vi "SC10_get_baud.vi"() -> ()   [LabVIEW 2010]
panel:
  out "substring":string
  in  "VISA resource name":refnum<visa-resource-name>
  out "VISA resource name out":refnum<visa-resource-name>
  out "read buffer":string
  out "return count 2":u32
  out "return count":u32
  out "error out":errorcluster
  in  "error in (no error)":errorcluster
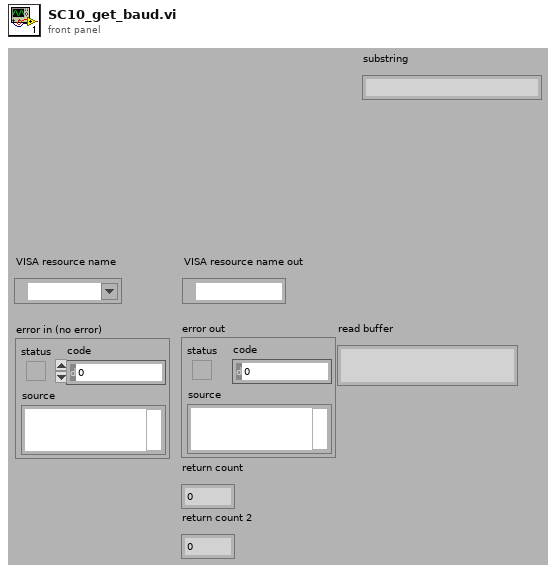
[diagram p1: front panel]
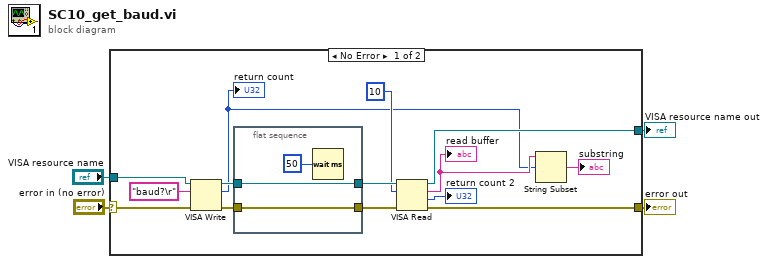
[diagram p0: block diagram]
diagram:
  n1 = case shown="No Error" "error in (no error)" {
    selector: "error in (no error)" -> [w14 w22]
    tunnel: [w13 w22] -> w3
    tunnel: [w9 w23] -> w2
    tunnel: "VISA resource name" -> [w8 w23]
    frame No Error {
      n2 = VISA Write(VISA resource name=w8, write buffer="baud?\r", error in (no error)=w14) -> (VISA resource name out=w18:refnum<visa-resource-name>, return count=w5:u32, error out=w16:errorcluster)
      "return count" <- w5
      n3 = flat-sequence {
        tunnel: w18 -> [w20]
        tunnel: [w20] -> w17
        tunnel: w16 -> [w19]
        tunnel: [w19] -> w15
        frame #0 {
          n4 = Wait (ms)(milliseconds to wait=u32 50) -> ()  [unwired: 1 out]
        }
      }
      n5 = VISA Read(VISA resource name=w17, byte count=u32 10, error in (no error)=w15) -> (VISA resource name out=w9:refnum<visa-resource-name>, read buffer=w7:string, return count=→"return count 2":u32, error out=w13:errorcluster)
      "read buffer" <- w7
      n6 = String Subset(string=w7, offset (0)=w5) -> (substring=→"substring":string)  [unwired: 1 in]
    }
    frame Error {
    }
  }
  "error out" <- w3
  "VISA resource name out" <- w2
